vi "Verificar conexão.vi"(8 "error in (no error)":errorcluster, 11 "Refnum in":T1) -> (0 "error out":errorcluster, 2 "Conectado":bool, 3 "Refnum out":T1)   [LabVIEW 2020, in "PostgreSQL Driver.lvlib"]
uses:
  <vilib>/addons/database/Connection.llb/Conn ObjectReference.ctl
  PostgreSQL Driver.lvlib
  <vilib>/addons/database/NI_Database_API.lvlib
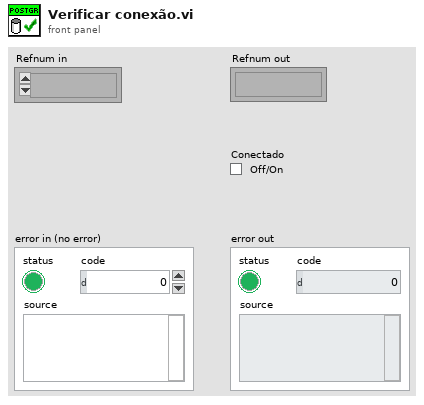
[diagram p1: front panel]
types:
  T1 = typedef "NI_Database_API.lvlib/Conn ObjectReference.ctl" = refnum<k1>
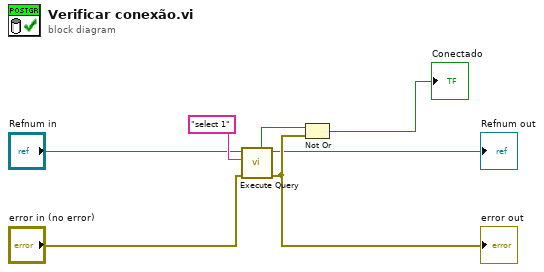
[diagram p0: block diagram]
diagram:
  n1 = call "Execute Query.vi"("error in (no error)"="error in (no error)", "SQL query"="select 1", "Connection in"="Refnum in") -> ("error out"=w7:errorcluster, "Connection out"=→"Refnum out":T1, "Sem dados?"=w6:bool)  [unwired: 4 in, 2 out]
  "error out" <- w7
  n2 = Not Or(1:w7, 2:w6) -> (0:→"Conectado":bool)
